vi "As xls format get data.vi"(9 "array size":i32, 11 "data in":string[](array[string])) -> (3 "result array":string[](array[string]))   [LabVIEW 2018]
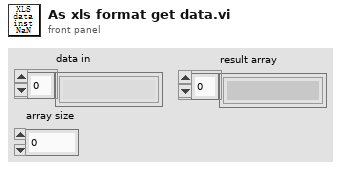
[diagram p1: front panel]
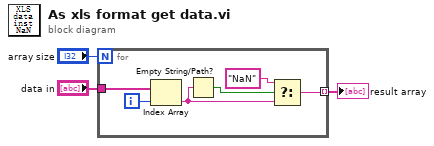
[diagram p0: block diagram]
diagram:
  n1 = for {
    N: "array size" -> [_]
    tunnel: "data in" -> [w6]
    tunnel: [w7] -> w1 mode=indexing
    i -> [w5]
    n2 = Index Array(array=w6, index=w5) -> (element=w4:string)
    n3 = Empty String/Path?(string/path=w4) -> (empty?=w9:bool)
    n4 = Select(t="NaN" ("字符串"), s=w9, f=w4) -> (s? t:f=w7:string)
  }
  "result array" <- w1
